vi "Finish.vi"   [LabVIEW 2013]
doc: "This VI is called just before exiting. It is expected to close I/O refnum, save collected data, etc."
uses:
  <vilib>/Rock Robotics/WPI/Joystick/WPI_JoystickGetSetRefNum.vi
  <vilib>/Rock Robotics/WPI/RobotDrive/WPI_RobotDriveGetSetRefNum.vi
  <vilib>/Rock Robotics/WPI/Compressor/WPI_CompressorGetSetRefNum.vi
types:
  T1 = typedef "WPI_AnalogChannelDevRef.ctl" = cluster{"DevStatus":errorcluster, "Analog Module":T2, "Analog Channel":T3}
  T2 = typedef "FPGA_TypedefAnalogModule.ctl" = enum16{"Analog Module 1", "Analog Module 2"}
  T3 = typedef "FPGA_AIChannel.ctl" = enum8{"AI 1", "AI 2", "AI 3", "AI 4", "AI 5", "AI 6", "AI 7", "AI 8", "Invalid"}
  T4 = typedef "WPI_CameraDevRef.ctl" = cluster{"Camera Address":string, "CameraStatus":errorcluster, "Acquire Image Notifier":refnum<notifier>}
  T5 = typedef "WPI_RobotDriveDevRef.ctl" = cluster{"DevStatus":errorcluster, "Motors[]":T6[], "Square Inputs":bool, "Max Output":dbl, "Isochronous":bool}
  T6 = typedef "WPI_MotorControlDeviceRef.ctl" = cluster{"DeviceStatus":errorcluster, "Type":enum16{"PWM", "CAN"}, "PWM":cluster{"Digital Module":T7, "PWM Channel":T8, "DeadBand":T9}, "CAN":cluster{"Device Number":u8, "Control Mode":T10, "Semaphore":T11, "Max Vout":dbl}, "Invert":bool, "TransformRef":T12, "InvTransformRef":T12}
  T7 = typedef "FPGA_TypedefDigitalModule.ctl" = enum16{"Digital Module 1", "Digital Module 2"}
  T8 = typedef "FPGA_DIOPWMChannel.ctl" = enum8{"PWM 1", "PWM 2", "PWM 3", "PWM 4", "PWM 5", "PWM 6", "PWM 7", "PWM 8", "PWM 9", "PWM 10", "Invalid"}
  T9 = typedef "WPI_PWMDeadband.ctl" = cluster{"Name":string, "maxPositivePwm":i32, "minPositivePwm":i32, "centerPwm":i32, "maxNegativePwm":i32, "minNegativePwm":i32, "angularRange":u16}
  T10 = typedef "WPI_CANJaguar_ControlMode.ctl" = enum8{"Percent VBus", "Current", "Speed", "Position", "Voltage"}
  T11 = typedef "Semaphore RefNum" = refnum<k1>
  T12 = typedef "WPI_PWMTransform_ConPane.ctl" = refnum<vi>
  T13 = typedef "WPI_ServoDeviceRef.ctl" = cluster{"DeviceStatus":errorcluster, "Digital Module":T7, "PWM Channel":T8, "DeadBand":T9}
  T14 = typedef "WPI_JoystickDevRef.ctl" = cluster{"Device":T15}
  T15 = typedef "WPI_JoystickDeviceEnum.ctl" = enum16{"USB 1", "USB 2", "USB 3", "USB 4", "Kinect 1", "Kinect 2"}
  T16 = typedef "WPI_DigitalInputDevRef.ctl" = cluster{"DevStatus":errorcluster, "DIO Channel":T17, "Digital Module":T7}
  T17 = typedef "FPGA_DIOChannel.ctl" = enum8{"DIO 1", "DIO 2", "DIO 3", "DIO 4", "DIO 5", "DIO 6", "DIO 7", "DIO 8", "DIO 9", "DIO 10", "DIO 11", "DIO 12", "DIO 13", "DIO 14", "Invalid"}
  T18 = typedef "WPI_SolenoidDevRef.ctl" = cluster{"DevStatus":errorcluster, "Solenoid Module":T19, "Forward Solenoid Channel":T20, "Reverse Solenoid Channel":T20}
  T19 = typedef "FPGA_TypedefSolenoidModule.ctl" = enum16{"Solenoid Module 1", "Solenoid Module 2"}
  T20 = typedef "WPI_SolenoidChannel.ctl" = enum8{"Solenoid 1", "Solenoid 2", "Solenoid 3", "Solenoid 4", "Solenoid 5", "Solenoid 6", "Solenoid 7", "Solenoid 8", "Invalid"}
  T21 = typedef "WPI_CompressorDevRef.ctl" = cluster{"DevStatus":errorcluster, "DigitalInputDevRef":T16, "RelayDevRef":T22}
  T22 = typedef "WPI_RelayDevRef.ctl" = cluster{"DevStatus":errorcluster, "Relay Channel":T23, "Digital Module":T7, "Relay Direction":T24}
  T23 = typedef "FPGA_DIORelayChannel.ctl" = enum8{"Relay 1", "Relay 2", "Relay 3", "Relay 4", "Relay 5", "Relay 6", "Relay 7", "Relay 8", "Invalid"}
  T24 = typedef "WPI_RelayDirection.ctl" = enum16{"Both directions", "Forward only", "Reverse only"}
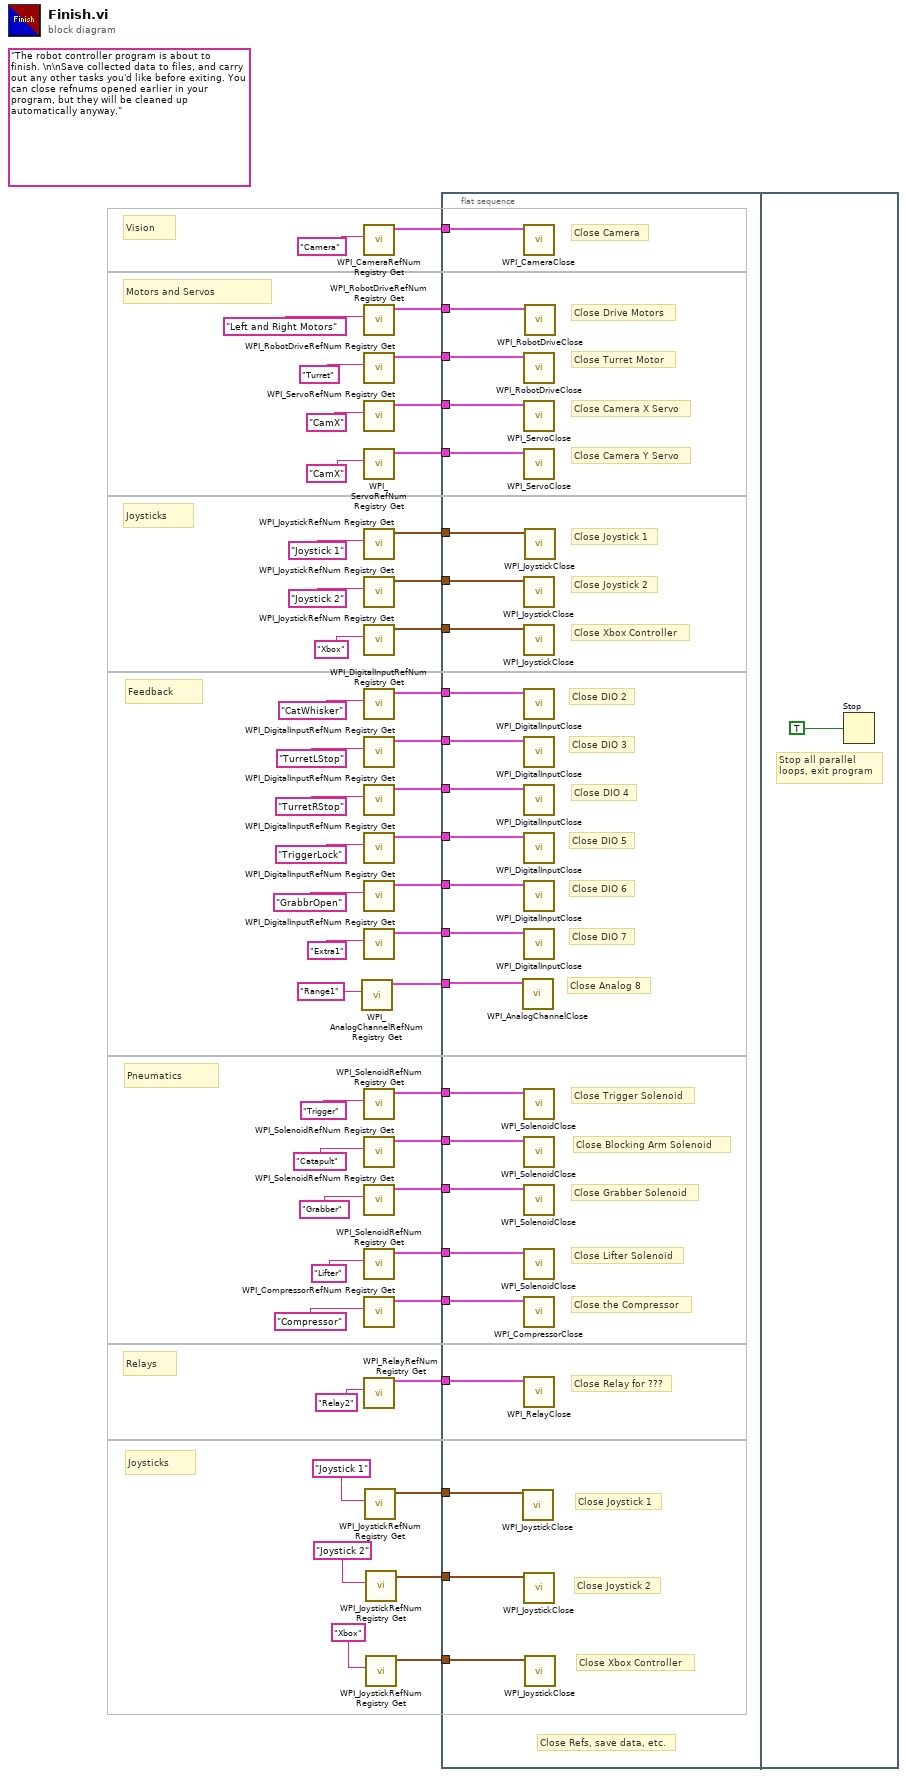
[diagram p0: block diagram]
diagram:
  (unwired) "The robot controller program is about to finish. \n\nSave collected data to files, and carry out any other tasks you'd like before exiting. You can close refnums opened earlier in your program, but they will be cleaned up automatically anyway."
  # "Joysticks"
  # "Joysticks"
  # "Relays"
  # "Pneumatics"
  # "Feedback"
  # "Motors and Servos"
  # "Vision"
  n1 = call <vilib>:"WPI_AnalogChannelRefNum Registry Get.vi"("refnum name"="Range1") -> ("AIDeviceRef"=w8:T1)  [unwired: 9 in, 1 out]
  n2 = call <vilib>:"WPI_CameraRefNum Registry Get.vi"("refnum name"="Camera") -> ("CameraDevRef"=w41:T4)  [unwired: 9 in, 1 out]
  n3 = call <vilib>:"WPI_RobotDriveRefNum Registry Get.vi"("refnum name"="Left and Right Motors") -> ("RobotDriveDevRef"=w46:T5)  [unwired: 1 in, 9 out]
  n4 = call <vilib>:"WPI_RobotDriveRefNum Registry Get.vi"("refnum name"="Turret") -> ("RobotDriveDevRef"=w10:T5)  [unwired: 1 in, 9 out]
  n5 = call <vilib>:"WPI_ServoRefNum Registry Get.vi"("refnum name"="CamX") -> ("ServoDeviceRef"=w25:T13)  [unwired: 9 in, 1 out]
  n6 = call <vilib>:"WPI_ServoRefNum Registry Get.vi"("refnum name"="CamX") -> ("ServoDeviceRef"=w24:T13)  [unwired: 9 in, 1 out]
  n7 = call <vilib>:"WPI_JoystickRefNum Registry Get.vi"("refnum name"="Joystick 1") -> ("JoystickDevRef"=w45:T14)  [unwired: 1 in, 9 out]
  n8 = call <vilib>:"WPI_JoystickRefNum Registry Get.vi"("refnum name"="Joystick 2") -> ("JoystickDevRef"=w43:T14)  [unwired: 1 in, 9 out]
  n9 = call <vilib>:"WPI_JoystickRefNum Registry Get.vi"("refnum name"="Xbox") -> ("JoystickDevRef"=w42:T14)  [unwired: 1 in, 9 out]
  n10 = call <vilib>:"WPI_DigitalInputRefNum Registry Get.vi"("refnum name"="CatWhisker") -> ("DigitalInputDevRef"=w30:T16)  [unwired: 9 in, 1 out]
  n11 = call <vilib>:"WPI_DigitalInputRefNum Registry Get.vi"("refnum name"="TurretLStop") -> ("DigitalInputDevRef"=w34:T16)  [unwired: 9 in, 1 out]
  n12 = call <vilib>:"WPI_DigitalInputRefNum Registry Get.vi"("refnum name"="TurretRStop") -> ("DigitalInputDevRef"=w33:T16)  [unwired: 9 in, 1 out]
  n13 = call <vilib>:"WPI_DigitalInputRefNum Registry Get.vi"("refnum name"="TriggerLock") -> ("DigitalInputDevRef"=w31:T16)  [unwired: 9 in, 1 out]
  n14 = call <vilib>:"WPI_DigitalInputRefNum Registry Get.vi"("refnum name"="GrabbrOpen") -> ("DigitalInputDevRef"=w32:T16)  [unwired: 9 in, 1 out]
  n15 = call <vilib>:"WPI_DigitalInputRefNum Registry Get.vi"("refnum name"="Extra1") -> ("DigitalInputDevRef"=w28:T16)  [unwired: 9 in, 1 out]
  n16 = call <vilib>:"WPI_SolenoidRefNum Registry Get.vi"("refnum name"="Trigger") -> ("SolenoidDevRef"=w21:T18)  [unwired: 9 in, 1 out]
  n17 = call <vilib>:"WPI_SolenoidRefNum Registry Get.vi"("refnum name"="Catapult") -> ("SolenoidDevRef"=w15:T18)  [unwired: 9 in, 1 out]
  n18 = call <vilib>:"WPI_SolenoidRefNum Registry Get.vi"("refnum name"="Grabber") -> ("SolenoidDevRef"=w17:T18)  [unwired: 9 in, 1 out]
  n19 = call <vilib>:"WPI_SolenoidRefNum Registry Get.vi"("refnum name"="Lifter") -> ("SolenoidDevRef"=w19:T18)  [unwired: 9 in, 1 out]
  n20 = call <vilib>:"WPI_CompressorRefNum Registry Get.vi"("refnum name"="Compressor") -> ("CompressorDevRef"=w14:T21)  [unwired: 9 in, 1 out]
  n21 = call <vilib>:"WPI_RelayRefNum Registry Get.vi"("refnum name"="Relay2") -> ("RelayDevRef"=w12:T22)  [unwired: 9 in, 1 out]
  n22 = call <vilib>:"WPI_JoystickRefNum Registry Get.vi"("refnum name"="Joystick 1") -> ("JoystickDevRef"=w4:T14)  [unwired: 9 in, 1 out]
  n23 = call <vilib>:"WPI_JoystickRefNum Registry Get.vi"("refnum name"="Joystick 2") -> ("JoystickDevRef"=w2:T14)  [unwired: 9 in, 1 out]
  n24 = call <vilib>:"WPI_JoystickRefNum Registry Get.vi"("refnum name"="Xbox") -> ("JoystickDevRef"=w1:T14)  [unwired: 9 in, 1 out]
  n25 = flat-sequence {
    tunnel: w46 -> [w72]
    tunnel: w45 -> [w71]
    tunnel: w43 -> [w70]
    tunnel: w42 -> [w69]
    tunnel: w41 -> [w68]
    tunnel: w34 -> [w67]
    tunnel: w33 -> [w66]
    tunnel: w32 -> [w65]
    tunnel: w31 -> [w64]
    tunnel: w30 -> [w63]
    tunnel: w28 -> [w62]
    tunnel: w25 -> [w61]
    tunnel: w24 -> [w60]
    tunnel: w21 -> [w58]
    tunnel: w19 -> [w57]
    tunnel: w17 -> [w56]
    tunnel: w15 -> [w55]
    tunnel: w14 -> [w59]
    tunnel: w12 -> [w54]
    tunnel: w10 -> [w53]
    tunnel: w8 -> [w52]
    tunnel: w4 -> [w51]
    tunnel: w2 -> [w50]
    tunnel: w1 -> [w49]
    frame #0 {
      # "Close Xbox Controller"
      # "Close Joystick 2"
      # "Close Joystick 1"
      # "Close Analog 8"
      # "Close Turret Motor"
      # "Close Relay for ???"
      # "Close the Compressor"
      # "Close Blocking Arm Solenoid"
      # "Close Grabber Solenoid"
      # "Close Lifter Solenoid"
      # "Close Trigger Solenoid"
      # "Close Camera Y Servo"
      # "Close Camera X Servo"
      # "Close DIO 7"
      # "Close DIO 2"
      # "Close DIO 5"
      # "Close DIO 6"
      # "Close DIO 4"
      # "Close DIO 3"
      # "Close Camera"
      # "Close Drive Motors"
      # "Close Xbox Controller"
      # "Close Joystick 2"
      # "Close Joystick 1"
      # "Close Refs, save data, etc."
      n26 = call <vilib>:"WPI_AnalogChannelClose.vi"("AIDeviceRef"=w52) -> ()  [unwired: 10 in, 1 out]
      n27 = call <vilib>:"WPI_JoystickClose.vi"("JoystickDevRef"=w51) -> ()  [unwired: 11 in]
      n28 = call <vilib>:"WPI_CameraClose.vi"("CameraDevRef"=w68) -> ()  [unwired: 10 in, 1 out]
      n29 = call <vilib>:"WPI_RobotDriveClose.vi"("RobotDriveDevRef"=w53) -> ()  [unwired: 1 in, 10 out]
      n30 = call <vilib>:"WPI_ServoClose.vi"("MotorControlDevRef"=w61) -> ()  [unwired: 10 in, 1 out]
      n31 = call <vilib>:"WPI_ServoClose.vi"("MotorControlDevRef"=w60) -> ()  [unwired: 10 in, 1 out]
      n32 = call <vilib>:"WPI_JoystickClose.vi"("JoystickDevRef"=w70) -> ()  [unwired: 11 out]
      n33 = call <vilib>:"WPI_JoystickClose.vi"("JoystickDevRef"=w69) -> ()  [unwired: 11 out]
      n34 = call <vilib>:"WPI_DigitalInputClose.vi"("DigitalInputDevRef"=w63) -> ()  [unwired: 10 in, 1 out]
      n35 = call <vilib>:"WPI_DigitalInputClose.vi"("DigitalInputDevRef"=w67) -> ()  [unwired: 10 in, 1 out]
      n36 = call <vilib>:"WPI_DigitalInputClose.vi"("DigitalInputDevRef"=w66) -> ()  [unwired: 10 in, 1 out]
      n37 = call <vilib>:"WPI_DigitalInputClose.vi"("DigitalInputDevRef"=w64) -> ()  [unwired: 10 in, 1 out]
      n38 = call <vilib>:"WPI_DigitalInputClose.vi"("DigitalInputDevRef"=w65) -> ()  [unwired: 10 in, 1 out]
      n39 = call <vilib>:"WPI_DigitalInputClose.vi"("DigitalInputDevRef"=w62) -> ()  [unwired: 10 in, 1 out]
      n40 = call <vilib>:"WPI_SolenoidClose.vi"("SolenoidDevRef"=w58) -> ()  [unwired: 10 in, 1 out]
      n41 = call <vilib>:"WPI_SolenoidClose.vi"("SolenoidDevRef"=w55) -> ()  [unwired: 10 in, 1 out]
      n42 = call <vilib>:"WPI_SolenoidClose.vi"("SolenoidDevRef"=w56) -> ()  [unwired: 10 in, 1 out]
      n43 = call <vilib>:"WPI_SolenoidClose.vi"("SolenoidDevRef"=w57) -> ()  [unwired: 10 in, 1 out]
      n44 = call <vilib>:"WPI_CompressorClose.vi"("CompressorDevRef"=w59) -> ()  [unwired: 10 in, 1 out]
      n45 = call <vilib>:"WPI_RelayClose.vi"("RelayDevRef"=w54) -> ()  [unwired: 10 in, 1 out]
      n46 = call <vilib>:"WPI_JoystickClose.vi"("JoystickDevRef"=w50) -> ()  [unwired: 11 in]
      n47 = call <vilib>:"WPI_RobotDriveClose.vi"("RobotDriveDevRef"=w72) -> ()  [unwired: 1 in, 10 out]
      n48 = call <vilib>:"WPI_JoystickClose.vi"("JoystickDevRef"=w71) -> ()  [unwired: 11 out]
      n49 = call <vilib>:"WPI_JoystickClose.vi"("JoystickDevRef"=w49) -> ()  [unwired: 11 in]
    }
    frame #1 {
      # "Stop all parallel\nloops, exit program"
      n50 = Stop(stop? (T)=TRUE ("Quit")) -> ()
    }
  }
